vi "PlayingSong.vi"(8 "error in (no error)":errorcluster, 10 "Message Queues in":T1, 11 "UI Refs":T2) -> (0 "error out":errorcluster, 2 "Message Queues out":T1, 3 "UI Refs out":T2)   [LabVIEW 2015]
uses:
  Controls & Type Defs/UI Data.ctl
  support/Message Queue/All Message Queues.ctl
  support/Message Queue/Message Cluster.ctl
  Controls & Type Defs/SongTimerModes.ctl
  support/Message Queue/Enqueue Message (Single).vi
  support/Message Queue/Message Queue.lvlib
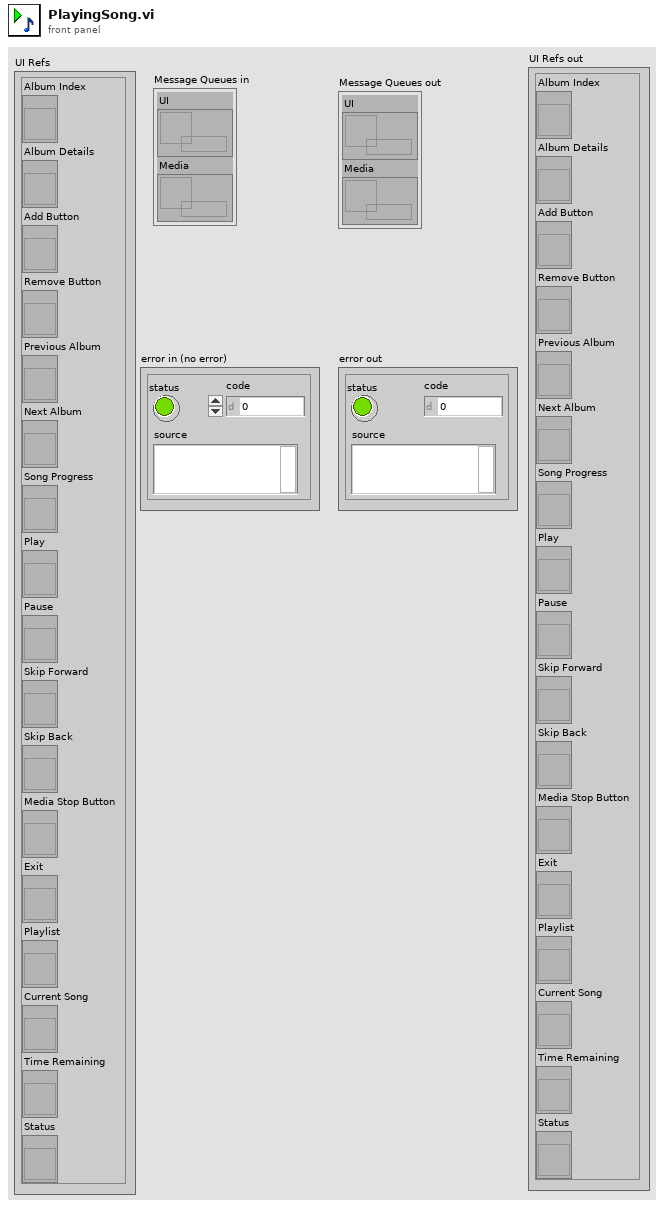
[diagram p1: front panel]
types:
  T1 = typedef "Message Queue.lvlib/All Message Queues.ctl" = cluster{"UI":refnum<queue>, "Media":refnum<queue>}
  T2 = typedef "UI Data.ctl" = cluster{"Album Index":refnum<vi>, "Album Details":refnum<vi>, "Add Button":refnum<vi>, "Remove Button":refnum<vi>, "Previous Album":refnum<vi>, "Next Album":refnum<vi>, "Song Progress":refnum<vi>, "Play":refnum<vi>, "Pause ":refnum<vi>, "Skip Forward":refnum<vi>, "Skip Back":refnum<vi>, "Media Stop Button":refnum<vi>, "Exit":refnum<vi>, "Playlist":refnum<vi>, "Current Song":refnum<vi>, "Time Remaining":refnum<vi>, "Status":refnum<vi>}
  T3 = typedef "SongTimerModes.ctl" = enum16{"Start", "Play", "Jump"}
  T4 = enum8{"Enabled", "Disabled", "Disabled and Grayed Out"}
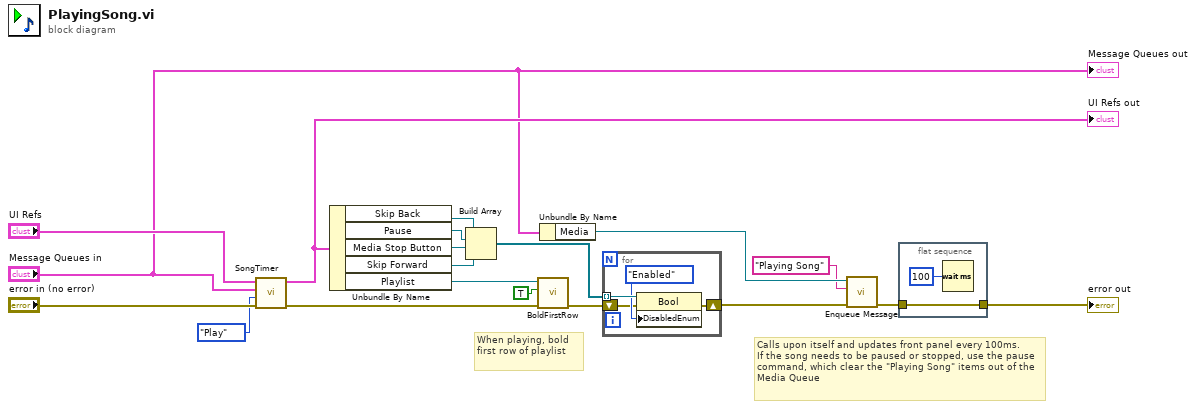
[diagram p0: block diagram]
diagram:
  # "When playing, bold first row of playlist"
  # "Calls upon itself and updates front panel every 100ms.\nIf the song needs to be paused or stopped, use the pause command, which clear the \"Playing Song\" items out of the Media Queue"
  n1 = call "SongTimer.vi"("error in (no error)"="error in (no error)", "Mode"=SongTimerModes."Play", "Message Queues in"="Message Queues in", "UI Refs in"="UI Refs") -> ("error out"=w4:errorcluster, "UI Refs out"=w15:T2)  [unwired: 6 in]
  "UI Refs out" <- w15
  n2 = Unbundle By Name(w15) -> ("Skip Back"=w19:refnum<vi>, "Pause"=w18:refnum<vi>, "Media Stop Button"=w17:refnum<vi>, "Skip Forward"=w16:refnum<vi>, "Playlist"=w3:refnum<vi>)
  n3 = Build Array(w19, w18, w17, w16) -> (w10:refnum<vi>[])
  n4 = call "BoldFirstRow.vi"("error in (no error)"=w4, "Bold first row?"=TRUE, "Playlist Ref"=w3) -> ("error out"=w2:errorcluster)  [unwired: 8 in]
  n5 = Unbundle By Name("Message Queues in") -> ("Media"=w8:refnum<queue>)
  n6 = for {
    tunnel: w10 -> [w23] mode=indexing
    shift-right: [w21] -> w5
    shift-left: w2 -> [w20]
    n7 = property class="Bool"(reference=w23, error in=w20, "DisabledEnum"=T4."Enabled" ("Disabled")) -> (error out=w21:errorcluster)  [unwired: 1 out]
  }
  n8 = call-poly "Enqueue Message.vi"("error in (no error)"=w5, "Message"="Playing Song", "Message Queue"=w8) -> ("error out"=w6:errorcluster)  [unwired: 7 in, 1 out]
  n9 = flat-sequence {
    tunnel: w6 -> [w24]
    tunnel: [w24] -> w14
    frame #0 {
      n10 = Wait (ms)(milliseconds to wait=u32 100) -> ()  [unwired: 1 out]
    }
  }
  "error out" <- w14
  "Message Queues out" <- "Message Queues in"
